vi "Revised-Math_Manipulation-16012016.vi"(6 "error in (no error)":errorcluster, 9 "Cluster":T1) -> (0 "error out":errorcluster, 2 "Final ODE":string[](array[string]), 3 "SP-for-ODE":string[](array[string]))   [LabVIEW 2014]
panel:
  out "R-Stoich-for ODE":string[](array[string])
  out "P-Stoich-for ODE":string[](array[string])
  out "P-Stoich-separate":string[](array[string])
  out "R-Stoich-separate":string[](array[string])
  out "Bound Cond ODE SP":string[](array[string])
  out "Sp_Id_Arr":string[](array[string])
  out "Bound Cond":string[](array[string])
  out "P-Stoich":string[](array[string])
  out "Kinetic Laws":string[](array[string])
  out "Products":string[](array[string])
  out "R-Stoich":string[](array[string])
  out "Reactants":string[](array[string])
  out "Intr_Kinetic_Law":string
  out "R-Sp-for-ODE":string[](array[string])
  out "P-SP-for-ODE":string[](array[string])
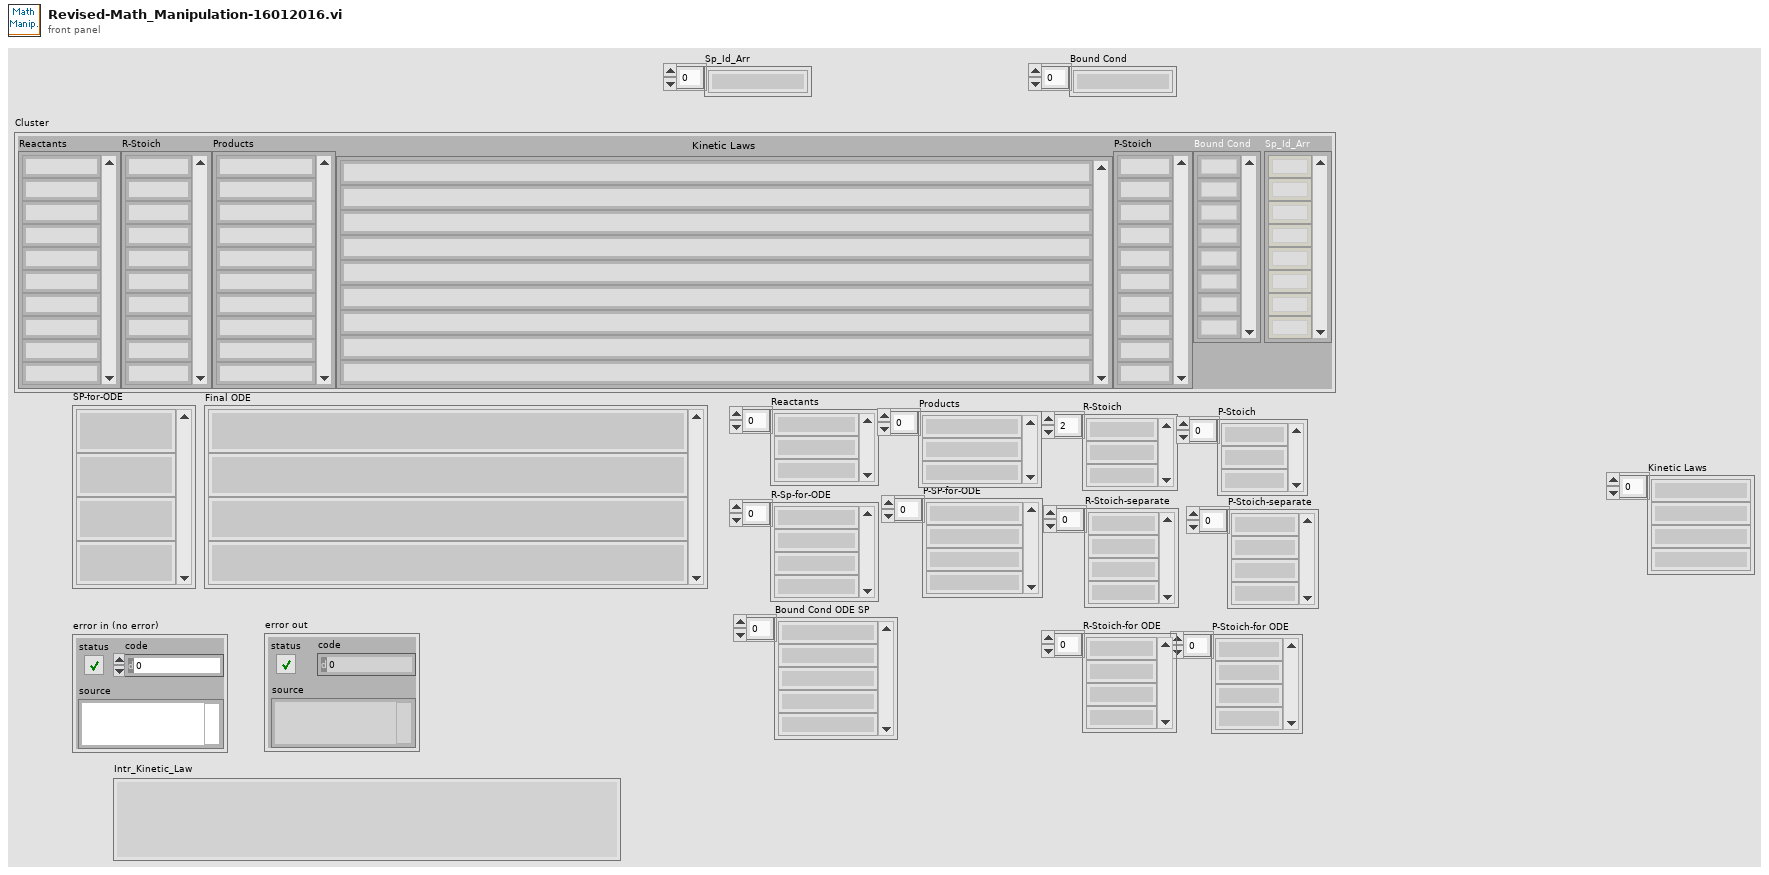
[diagram p1: front panel]
types:
  T1 = cluster{"Reactants":string[], "R-Stoich":string[], "Products":string[], "Kinetic Laws":string[], "P-Stoich":string[], "Bound Cond":string[], "Sp_Id_Arr":string[]}
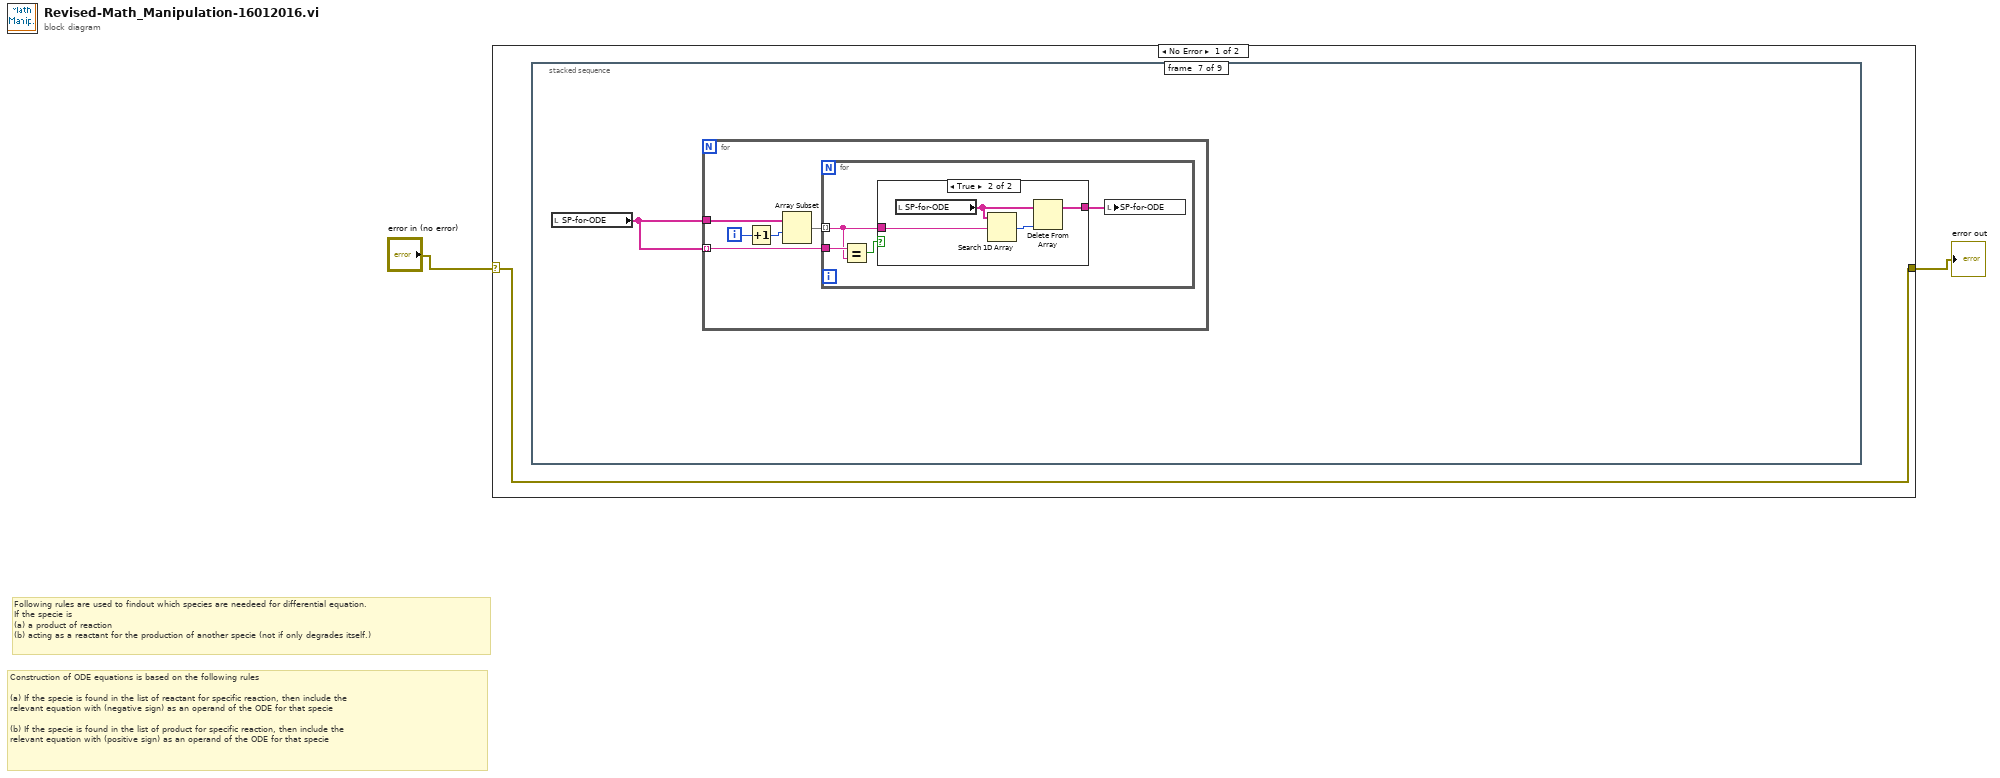
[diagram p0: block diagram]
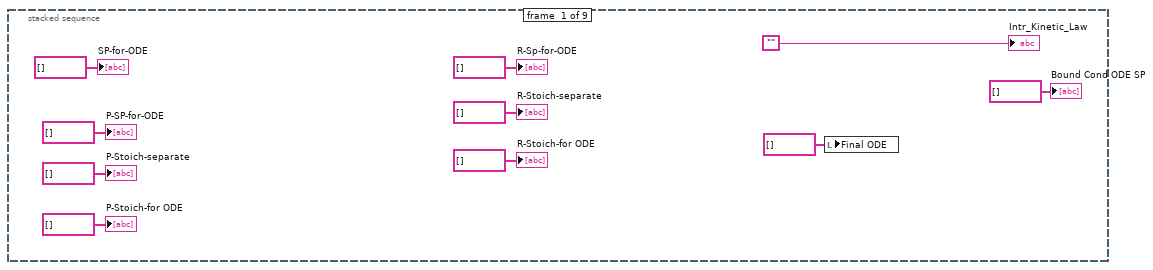
[diagram p2: hidden frame]
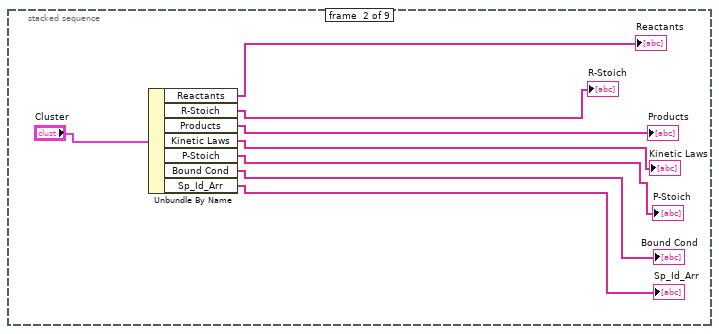
[diagram p3: hidden frame]
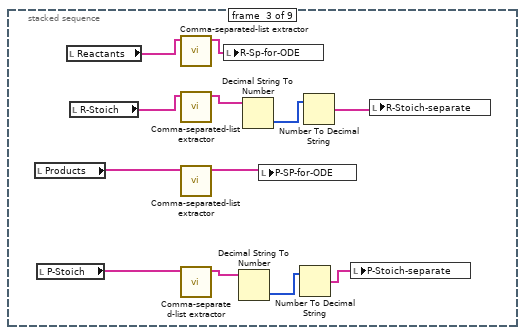
[diagram p4: hidden frame]
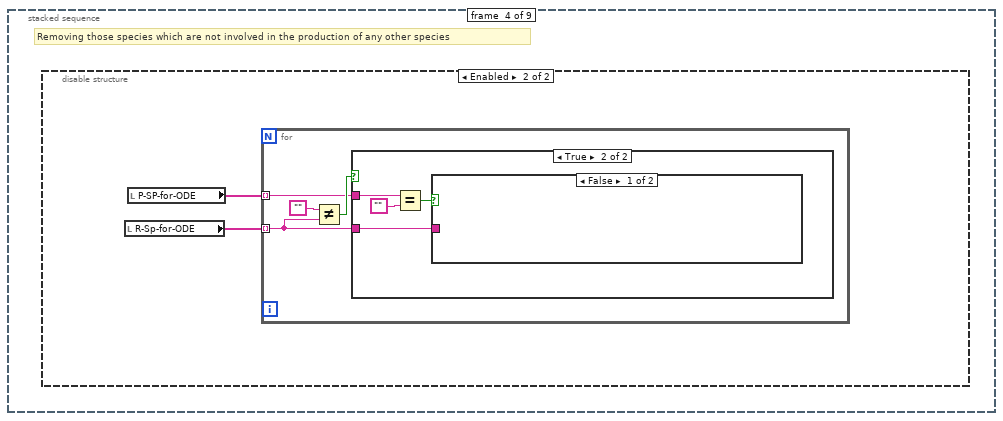
[diagram p5: hidden frame]
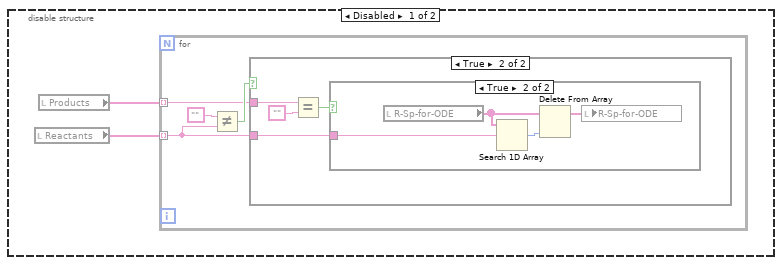
[diagram p6: hidden frame]
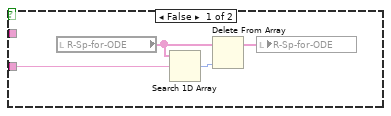
[diagram p7: hidden frame]
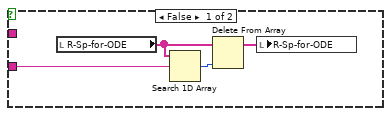
[diagram p9: hidden frame]
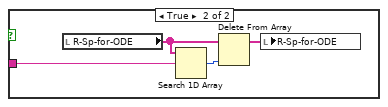
[diagram p10: hidden frame]
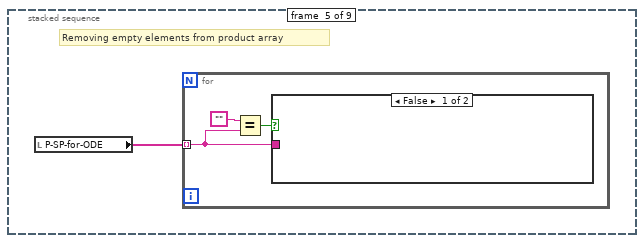
[diagram p11: hidden frame]
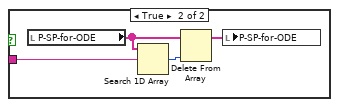
[diagram p12: hidden frame]
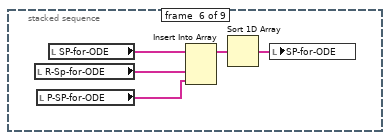
[diagram p13: hidden frame]
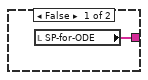
[diagram p14: hidden frame]
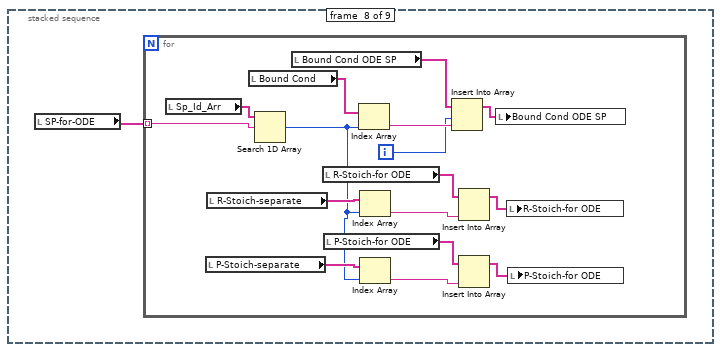
[diagram p15: hidden frame]
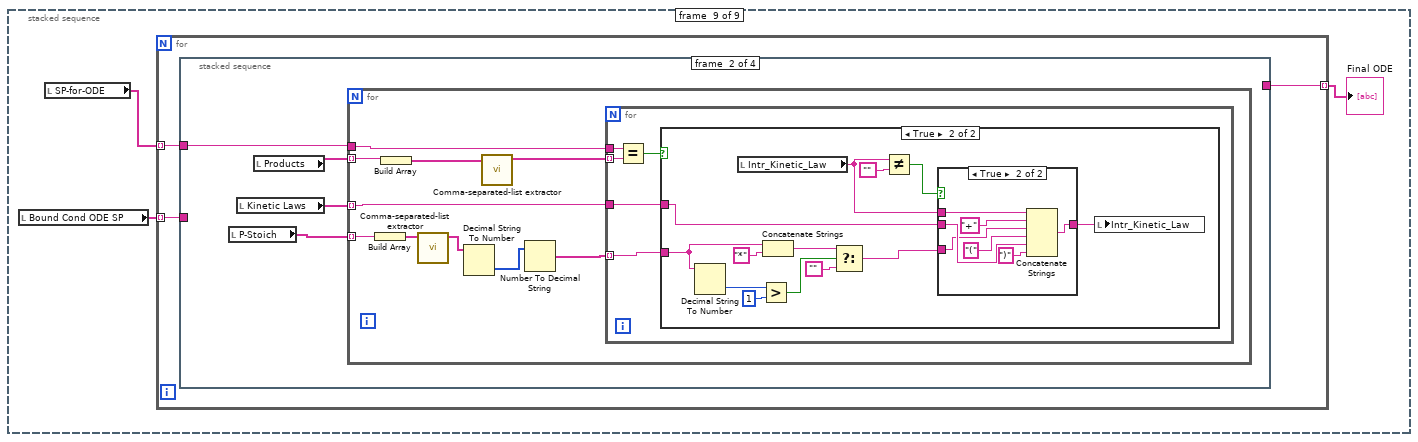
[diagram p16: hidden frame]
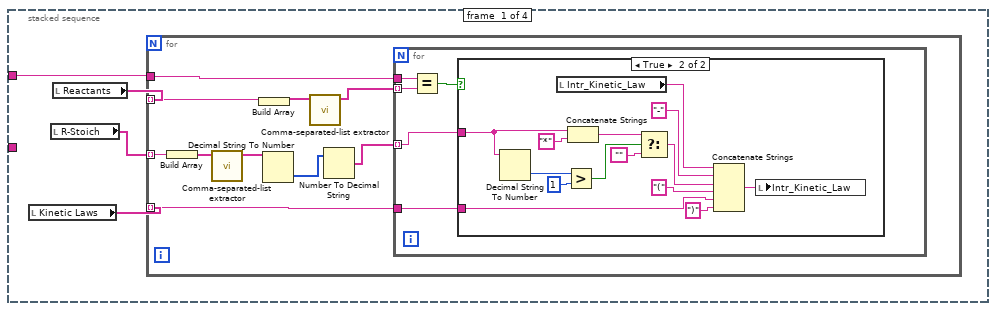
[diagram p17: hidden frame]
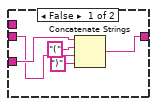
[diagram p20: hidden frame]
diagram:
  # "Construction of ODE equations is based on the following rules\n\n(a) If the specie is found in the list of reactant for specific reaction, then include the \nrelevant equation with (negative sign) as an operand of the ODE for that specie\n\n(b) If the specie is found in the list of product for specific reaction, then include the \nrelevant equation with (positive sign) as an operand of the ODE for that specie"
  # "Following rules are used to findout which species are needeed for differential equation.\nIf the specie is \n(a) a product of reaction\n(b) acting as a reactant for the production of another specie (not if only degrades itself.)"
  n1 = case shown="No Error" "error in (no error)" {
    selector: "error in (no error)" -> [w3 w205]
    tunnel: [w3 w205] -> w1
    frame No Error {
      n2 = stacked-sequence {
        frame #0 {
          n3 = local write "Final ODE"(string[] [] ("Final ODE")) -> ()
          "SP-for-ODE" <- string[] [] ("output array")
          "P-SP-for-ODE" <- string[] [] ("output array")
          "R-Sp-for-ODE" <- string[] [] ("output array")
          "Intr_Kinetic_Law" <- ""
          "Bound Cond ODE SP" <- string[] [] ("Bound Cond ODE SP")
          "R-Stoich-separate" <- string[] [] ("output array")
          "P-Stoich-separate" <- string[] [] ("output array")
          "P-Stoich-for ODE" <- string[] [] ("output array")
          "R-Stoich-for ODE" <- string[] [] ("output array")
        }
        frame #1 {
          n4 = Unbundle By Name("Cluster") -> ("Reactants"=→"Reactants":string[], "R-Stoich"=→"R-Stoich":string[], "Products"=→"Products":string[], "Kinetic Laws"=→"Kinetic Laws":string[], "P-Stoich"=→"P-Stoich":string[], "Bound Cond"=→"Bound Cond":string[], "Sp_Id_Arr"=→"Sp_Id_Arr":string[])
        }
        frame #2 {
          n5 = local read "Products"() -> (w27:string[])
          n6 = local read "P-Stoich"() -> (w25:string[])
          n7 = local read "Reactants"() -> (w33:string[])
          n8 = local read "R-Stoich"() -> (w31:string[])
          n9 = call "Comma-separated-list extractor.vi"("In_list"=w33) -> ("List_Out"=w32:string[])  [unwired: 6 in, 1 out]
          n10 = call "Comma-separated-list extractor.vi"("In_list"=w31) -> ("List_Out"=w29:string[])  [unwired: 6 in, 1 out]
          n11 = call "Comma-separated-list extractor.vi"("In_list"=w27) -> ("List_Out"=w26:string[])  [unwired: 6 in, 1 out]
          n12 = call "Comma-separated-list extractor.vi"("In_list"=w25) -> ("List_Out"=w23:string[])  [unwired: 6 in, 1 out]
          n13 = local write "R-Sp-for-ODE"(w32) -> ()
          n14 = Decimal String To Number(string=w23) -> (number=w24:i32[])  [unwired: 2 in, 1 out]
          n15 = Decimal String To Number(string=w29) -> (number=w30:i32[])  [unwired: 2 in, 1 out]
          n16 = local write "P-SP-for-ODE"(w26) -> ()
          n17 = Number To Decimal String(number=w24) -> (decimal integer string=w22:string[])  [unwired: 1 in]
          n18 = Number To Decimal String(number=w30) -> (decimal integer string=w28:string[])  [unwired: 1 in]
          n19 = local write "P-Stoich-separate"(w22) -> ()
          n20 = local write "R-Stoich-separate"(w28) -> ()
        }
        frame #3 {
          # "Removing those species which are not involved in the production of any other species"
          n21 = disable-structure shown="Enabled" {
            frame Disabled {
              n22 = local read "Reactants"() -> (w35:string[])
              n23 = local read "Products"() -> (w34:string[])
              n24 = for {
                tunnel: w35 -> [w36] mode=indexing
                tunnel: w34 -> [w38] mode=indexing
                n25 = Not Equal?(x="", y=w36) -> (x != y?=w39:bool)
                n26 = case shown="True" w39 {
                  tunnel: w38 -> [_ w46]
                  tunnel: w36 -> [w40 w44]
                  frame False {
                    n27 = local read "R-Sp-for-ODE"() -> (w43:string[])
                    n28 = Search 1D Array(1D array=w43, element=w40) -> (index of element=w42:i32)  [unwired: 1 in]
                    n29 = Delete From Array(array=w43, index=w42) -> (array with subset deleted=w41:string[])  [unwired: 1 in, 1 out]
                    n30 = local write "R-Sp-for-ODE"(w41) -> ()
                  }
                  frame True {
                    n31 = Equal?(x=w46, y="") -> (x = y?=w45:bool)
                    n32 = case shown="True" w45 {
                      tunnel: w44 -> [_ w51]
                      frame False {
                      }
                      frame True {
                        n33 = local read "R-Sp-for-ODE"() -> (w50:string[])
                        n34 = Search 1D Array(1D array=w50, element=w51) -> (index of element=w49:i32)  [unwired: 1 in]
                        n35 = Delete From Array(array=w50, index=w49) -> (array with subset deleted=w48:string[])  [unwired: 1 in, 1 out]
                        n36 = local write "R-Sp-for-ODE"(w48) -> ()
                      }
                    }
                  }
                }
              }
            }
            frame Enabled {
              n37 = local read "R-Sp-for-ODE"() -> (w53:string[])
              n38 = local read "P-SP-for-ODE"() -> (w52:string[])
              n39 = for {
                tunnel: w53 -> [w54] mode=indexing
                tunnel: w52 -> [w56] mode=indexing
                n40 = Not Equal?(x="", y=w54) -> (x != y?=w57:bool)
                n41 = case shown="True" w57 {
                  tunnel: w56 -> [_ w64]
                  tunnel: w54 -> [w58 w62]
                  frame False {
                    n42 = local read "R-Sp-for-ODE"() -> (w61:string[])
                    n43 = Search 1D Array(1D array=w61, element=w58) -> (index of element=w60:i32)  [unwired: 1 in]
                    n44 = Delete From Array(array=w61, index=w60) -> (array with subset deleted=w59:string[])  [unwired: 1 in, 1 out]
                    n45 = local write "R-Sp-for-ODE"(w59) -> ()
                  }
                  frame True {
                    n46 = Equal?(x=w64, y="") -> (x = y?=w63:bool)
                    n47 = case shown="False" w63 {
                      tunnel: w62 -> [_ w69]
                      frame False {
                      }
                      frame True {
                        n48 = local read "R-Sp-for-ODE"() -> (w68:string[])
                        n49 = Search 1D Array(1D array=w68, element=w69) -> (index of element=w67:i32)  [unwired: 1 in]
                        n50 = Delete From Array(array=w68, index=w67) -> (array with subset deleted=w66:string[])  [unwired: 1 in, 1 out]
                        n51 = local write "R-Sp-for-ODE"(w66) -> ()
                      }
                    }
                  }
                }
              }
            }
          }
        }
        frame #4 {
          # "Removing empty elements from product array"
          n52 = local read "P-SP-for-ODE"() -> (w70:string[])
          n53 = for {
            tunnel: w70 -> [w71] mode=indexing
            n54 = Equal?(x="", y=w71) -> (x = y?=w72:bool)
            n55 = case shown="False" w72 {
              tunnel: w71 -> [_ w77]
              frame False {
              }
              frame True {
                n56 = local read "P-SP-for-ODE"() -> (w76:string[])
                n57 = Search 1D Array(1D array=w76, element=w77) -> (index of element=w75:i32)  [unwired: 1 in]
                n58 = Delete From Array(array=w76, index=w75) -> (array with subset deleted=w74:string[])  [unwired: 1 in, 1 out]
                n59 = local write "P-SP-for-ODE"(w74) -> ()
              }
            }
          }
        }
        frame #5 {
          n60 = local read "R-Sp-for-ODE"() -> (w81:string[])
          n61 = local read "P-SP-for-ODE"() -> (w80:string[])
          n62 = local read "SP-for-ODE"() -> (w82:string[])
          n63 = Insert Into Array(array=w82, new element #1=w81, new element #2=w80) -> (w79:string[])  [unwired: 1 in]
          n64 = Sort 1D Array(array=w79) -> (sorted array=w78:string[])
          n65 = local write "SP-for-ODE"(w78) -> ()
        }
        frame #6 {
          n66 = local read "SP-for-ODE"() -> (w83:string[])
          n67 = for {
            tunnel: w83 -> [w85] mode=indexing
            tunnel: w83 -> [w88]
            i -> [w84]
            n68 = Increment(x=w84) -> (x+1=w87:i32)
            n69 = Array Subset(array=w88, index=w87) -> (w86:string[])  [unwired: 1 in]
            n70 = for {
              tunnel: w86 -> [w89] mode=indexing
              tunnel: w85 -> [w92]
              n71 = Equal?(x=w92, y=w89) -> (x = y?=w91:bool)
              n72 = case shown="True" w91 {
                tunnel: [w93 w97] -> w90
                tunnel: w89 -> [_ w94]
                frame False {
                  n73 = local read "SP-for-ODE"() -> (w93:string[])
                }
                frame True {
                  n74 = local read "SP-for-ODE"() -> (w96:string[])
                  n75 = Search 1D Array(1D array=w96, element=w94) -> (index of element=w95:i32)  [unwired: 1 in]
                  n76 = Delete From Array(array=w96, index=w95) -> (array with subset deleted=w97:string[])  [unwired: 1 in, 1 out]
                }
              }
              n77 = local write "SP-for-ODE"(w90) -> ()
            }
          }
        }
        frame #7 {
          n78 = local read "SP-for-ODE"() -> (w98:string[])
          n79 = for {
            tunnel: w98 -> [w113] mode=indexing
            i -> [w108]
            n80 = local read "Sp_Id_Arr"() -> (w114:string[])
            n81 = local read "P-Stoich-separate"() -> (w100:string[])
            n82 = local read "R-Stoich-separate"() -> (w107:string[])
            n83 = local read "Bound Cond"() -> (w112:string[])
            n84 = Search 1D Array(1D array=w114, element=w113) -> (index of element=w99:i32)  [unwired: 1 in]
            n85 = local read "Bound Cond ODE SP"() -> (w109:string[])
            n86 = local read "R-Stoich-for ODE"() -> (w105:string[])
            n87 = local read "P-Stoich-for ODE"() -> (w102:string[])
            n88 = Index Array(array=w112, index=w99) -> (element=w111:string)
            n89 = Index Array(array=w107, index=w99) -> (element=w106:string)
            n90 = Index Array(array=w100, index=w99) -> (element=w101:string)
            n91 = Insert Into Array(array=w109, index=w108, new element=w111) -> (w110:string[])
            n92 = Insert Into Array(array=w105, new element=w106) -> (w104:string[])  [unwired: 1 in]
            n93 = Insert Into Array(array=w102, new element=w101) -> (w103:string[])  [unwired: 1 in]
            n94 = local write "Bound Cond ODE SP"(w110) -> ()
            n95 = local write "R-Stoich-for ODE"(w104) -> ()
            n96 = local write "P-Stoich-for ODE"(w103) -> ()
          }
        }
        frame #8 {
          n97 = local read "Bound Cond ODE SP"() -> (w115:string[])
          n98 = local read "SP-for-ODE"() -> (w117:string[])
          n99 = for {
            tunnel: w117 -> [w120] mode=indexing
            tunnel: [w119] -> w116 mode=indexing
            tunnel: w115 -> [w118] mode=indexing
            n100 = stacked-sequence {
              tunnel: w120 -> [w124 w156 _ _]
              tunnel: [_ _ w200 _] -> w119
              tunnel: w118 -> [_ _ w201 _]
              frame #0 {
                n101 = local read "Kinetic Laws"() -> (w123:string[])
                n102 = local read "R-Stoich"() -> (w121:string[])
                n103 = local read "Reactants"() -> (w122:string[])
                n104 = for {
                  tunnel: w124 -> [w134]
                  tunnel: w123 -> [w133] mode=indexing
                  tunnel: w122 -> [w130] mode=indexing
                  tunnel: w121 -> [w127] mode=indexing
                  n105 = Build Array(w127) -> (w126:string[])
                  n106 = call "Comma-separated-list extractor.vi"("In_list"=w126) -> ("List_Out"=w125:string[])  [unwired: 6 in, 1 out]
                  n107 = Build Array(w130) -> (w129:string[])
                  n108 = Decimal String To Number(string=w125) -> (number=w132:i32[])  [unwired: 2 in, 1 out]
                  n109 = call "Comma-separated-list extractor.vi"("In_list"=w129) -> ("List_Out"=w128:string[])  [unwired: 6 in, 1 out]
                  n110 = Number To Decimal String(number=w132) -> (decimal integer string=w131:string[])  [unwired: 1 in]
                  n111 = for {
                    tunnel: w134 -> [w139]
                    tunnel: w128 -> [w138] mode=indexing
                    tunnel: w133 -> [w136]
                    tunnel: w131 -> [w135] mode=indexing
                    n112 = Equal?(x=w139, y=w138) -> (x = y?=w137:bool)
                    n113 = case shown="True" w137 {
                      tunnel: w135 -> [_ w145]
                      tunnel: w136 -> [_ w140]
                      frame False {
                      }
                      frame True {
                        n114 = Decimal String To Number(string=w145) -> (number=w148:i32)  [unwired: 2 in, 1 out]
                        n115 = local read "Intr_Kinetic_Law"() -> (w149:string)
                        n116 = Greater?(x=w148, y=1) -> (0:w146:bool)
                        n117 = Concatenate Strings(w145, "*" ("string")) -> (w143:string)
                        n118 = Select(t=w143, s=w146, f="") -> (s? t:f=w142:string)
                        n119 = Concatenate Strings(w149, "-" ("string"), w142, "(" ("string"), w140, ")" ("string")) -> (w150:string)
                        n120 = local write "Intr_Kinetic_Law"(w150) -> ()
                      }
                    }
                  }
                }
              }
              frame #1 {
                n121 = local read "P-Stoich"() -> (w155:string[])
                n122 = local read "Kinetic Laws"() -> (w154:string[])
                n123 = local read "Products"() -> (w157:string[])
                n124 = for {
                  tunnel: w157 -> [w161] mode=indexing
                  tunnel: w156 -> [w167]
                  tunnel: w155 -> [w158] mode=indexing
                  tunnel: w154 -> [w166] mode=indexing
                  n125 = Build Array(w158) -> (w159:string[])
                  n126 = Build Array(w161) -> (w160:string[])
                  n127 = call "Comma-separated-list extractor.vi"("In_list"=w159) -> ("List_Out"=w163:string[])  [unwired: 6 in, 1 out]
                  n128 = Decimal String To Number(string=w163) -> (number=w164:i32[])  [unwired: 2 in, 1 out]
                  n129 = call "Comma-separated-list extractor.vi"("In_list"=w160) -> ("List_Out"=w165:string[])  [unwired: 6 in, 1 out]
                  n130 = Number To Decimal String(number=w164) -> (decimal integer string=w162:string[])  [unwired: 1 in]
                  n131 = for {
                    tunnel: w167 -> [w172]
                    tunnel: w165 -> [w171] mode=indexing
                    tunnel: w162 -> [w169] mode=indexing
                    tunnel: w166 -> [w168]
                    n132 = Equal?(x=w172, y=w171) -> (x = y?=w170:bool)
                    n133 = case shown="True" w170 {
                      tunnel: w169 -> [_ w174]
                      tunnel: w168 -> [_ w173]
                      frame False {
                      }
                      frame True {
                        n134 = Decimal String To Number(string=w174) -> (number=w181:i32)  [unwired: 2 in, 1 out]
                        n135 = local read "Intr_Kinetic_Law"() -> (w183:string)
                        n136 = Greater?(x=w181, y=1) -> (0:w179:bool)
                        n137 = Concatenate Strings(w174, "*" ("string")) -> (w177:string)
                        n138 = Select(t=w177, s=w179, f="") -> (s? t:f=w175:string)
                        n139 = Not Equal?(x=w183, y="") -> (x != y?=w182:bool)
                        n140 = case shown="True" w182 {
                          tunnel: w173 -> [w188 w194]
                          tunnel: [w187 w193] -> w185
                          tunnel: w183 -> [_ w192]
                          tunnel: w175 -> [w189 w191]
                          frame False {
                            n141 = Concatenate Strings(w189, "(" ("string"), w188, ")" ("string")) -> (w187:string)
                          }
                          frame True {
                            n142 = Concatenate Strings(w192, "+" ("string"), w191, "(" ("string"), w194, ")" ("string")) -> (w193:string)
                          }
                        }
                        n143 = local write "Intr_Kinetic_Law"(w185) -> ()
                      }
                    }
                  }
                }
              }
              frame #2 {
                n144 = Equal?(x=w201, y="false") -> (x = y?=w198:bool)
                n145 = case shown="True" w198 {
                  tunnel: ["" w203] -> w200
                  frame False {
                  }
                  frame True {
                    n146 = local read "Intr_Kinetic_Law"() -> (w203:string)
                  }
                }
              }
              frame #3 {
                n147 = local write "Intr_Kinetic_Law"("") -> ()
              }
            }
          }
          "Final ODE" <- w116
        }
      }
    }
    frame Error {
    }
  }
  "error out" <- w1
